vi "Read Non-Sequential Address.vi"(7 "Target IC (1-8)":u8, 8 "error in (no error)":errorcluster, 10 "Address":u16 format="%04x", 11 "FPGA Interface in":refnum<class "FPGA Interface.lvclass">) -> (0 "error out":errorcluster, 2 "Data":u16 format="%04x")   [LabVIEW 2020, in "BCI-1553 API.lvlib" / "FPGA Interface.lvlib" / "FPGA Interface.lvclass"]
doc: "Reads an arbitrary address from a component in the 1553 Session. This method blocks until it receives data back from the specified component."
uses:
  FPGA Interface.lvclass
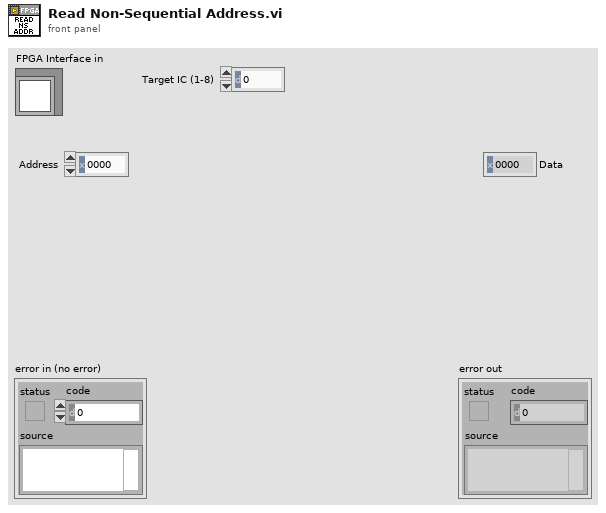
[diagram p1: front panel]
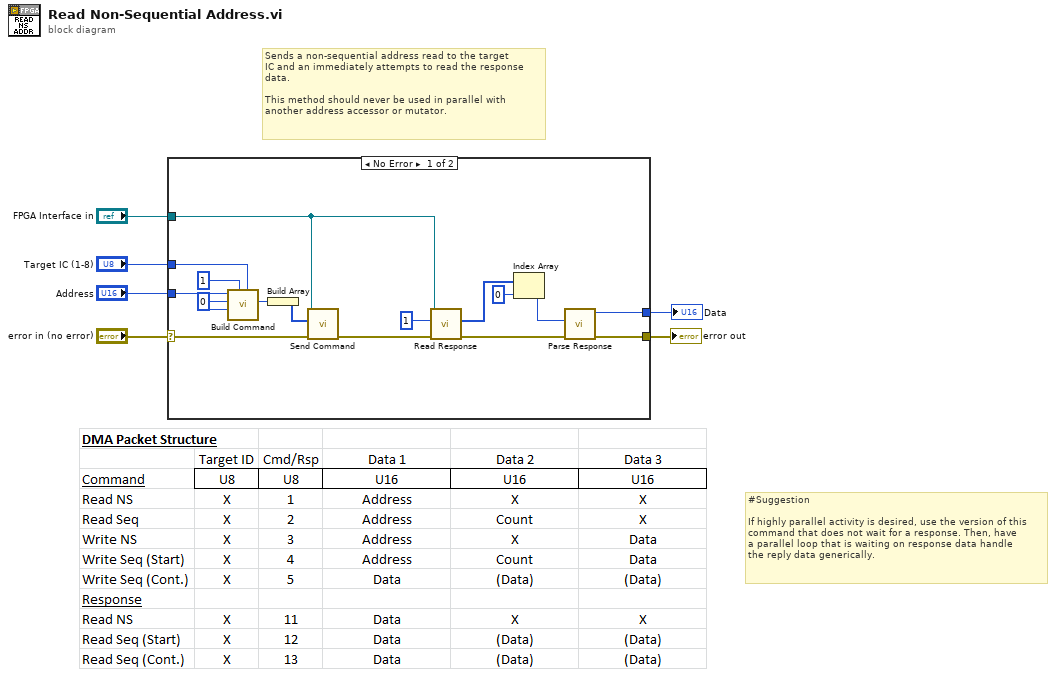
[diagram p0: block diagram]
diagram:
  # "#Suggestion\n\nIf highly parallel activity is desired, use the version of this\ncommand that does not wait for a response. Then, have\na parallel loop that is waiting on response data handle\nthe reply data generically."
  # "Sends a non-sequential address read to the target\nIC and an immediately attempts to read the response\ndata.\n\nThis method should never be used in parallel with\nanother address accessor or mutator."
  n1 = case shown="No Error" "error in (no error)" {
    selector: "error in (no error)" -> [w19 w23]
    tunnel: [w10 w23] -> w5
    tunnel: "FPGA Interface in" -> [w18 _]
    tunnel: "Target IC (1-8)" -> [w9 _]
    tunnel: "Address" -> [w22 _]
    tunnel: [w11 _] -> w1
    frame No Error {
      w7 = u16 0 ("Data 2")
      n2 = call "Build Command.vi"("Target"=w9, "CMD ID"=u8 1, "Data 3"=w7, "Data 2"=w7, "Data 1"=w22) -> ("Command"=w21:u64)  [unwired: 5 in, 1 out]
      n3 = Build Array(w21) -> (w20:u64[])
      n4 = call "Send Command.vi"("error in (no error)"=w19, "Data"=w20, "FPGA Interface in"=w18) -> ("error out"=w16:errorcluster)  [unwired: 8 in]
      n5 = call "Read Response.vi"("error in (no error)"=w16, "Number of Elements"=u32 1, "FPGA Interface in"=w18) -> ("error out"=w15:errorcluster, "Data"=w14:u64[])  [unwired: 6 in, 1 out]
      n6 = Index Array(array=w14, index=0) -> (element=w12:u64)
      n7 = call "Parse Response.vi"("error in (no error)"=w15, "Data"=w12) -> ("error out"=w10:errorcluster, "Data 1"=w11:u16)  [unwired: 4 in, 4 out]
    }
    frame Error {
    }
  }
  "error out" <- w5
  "Data" <- w1
